vi "4155C Make Big 2d array FPP.vi"(0 "1D Var1":dbl[](array[numeric])=[0.0, 1.0, 2.0, 3.0, 4.0, 5.0, 6.0, 7.0, 8.0, 9.0, 10.0, 11.0] format="%.2f", 2 "1d ID":dbl[](array[numeric])=[20.0, 21.0, 22.0, 23.0, 24.0, 25.0, 26.0, 27.0, 28.0, 29.0, 30.0, 31.0] format="%.2f", 3 "1d Vp2":dbl[](array[numeric])=[20.0, 21.0, 22.0, 23.0, 24.0, 25.0, 26.0, 27.0, 28.0, 29.0, 30.0, 31.0] format="%.2f", 4 "1d IG":dbl[](array[numeric])=[40.0, 41.0, 42.0, 43.0, 44.0, 45.0, 46.0, 47.0, 48.0, 49.0, 50.0, 51.0] format="%.2f", 6 "1d Vp1":dbl[](array[numeric])=[60.0, 61.0, 62.0, 63.0, 64.0, 65.0, 66.0, 67.0, 68.0, 69.0, 70.0, 71.0] format="%.2f", 10 "VAR2 START":dbl format="%.2f", 11 "Number of VAR2 steps":i32=6, 14 "VAR2 STEP":dbl format="%.2f", 15 "VAR1 Name":string, 24 "Decimal places in header":i8=1, 26 "VAR2 Name":string) -> (20 "Header array":string[](array[string]), 22 "Data array":dbl[][](array[numeric]) format="%.2f")   [LabVIEW 2019]
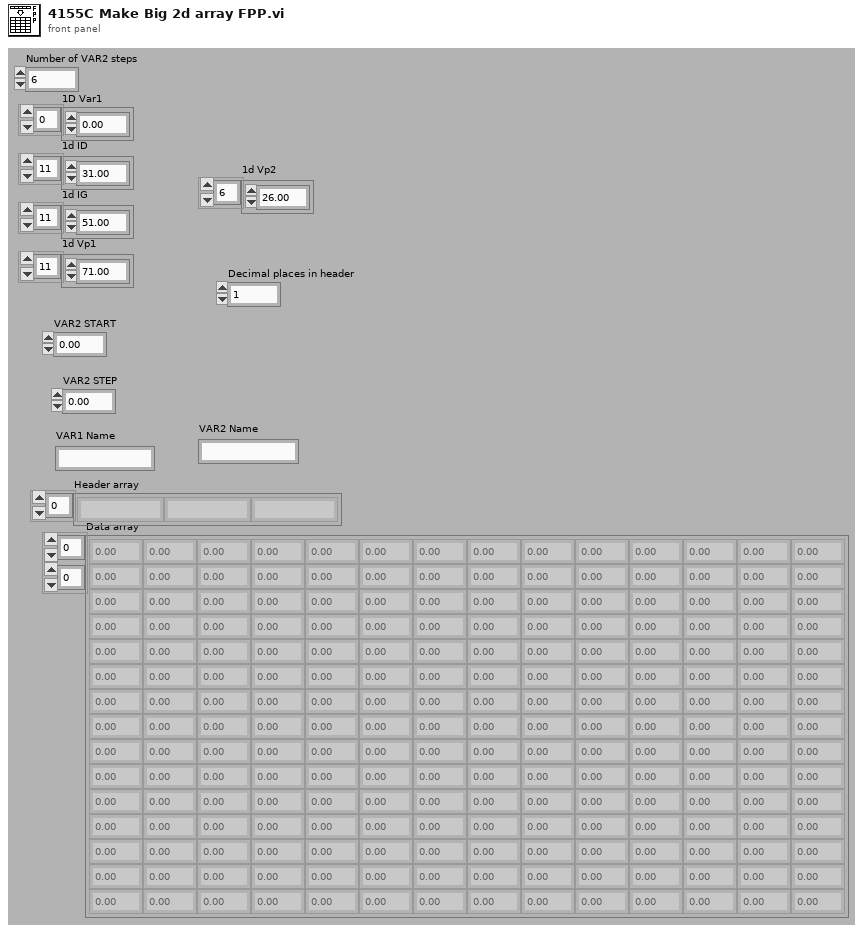
[diagram p1: front panel]
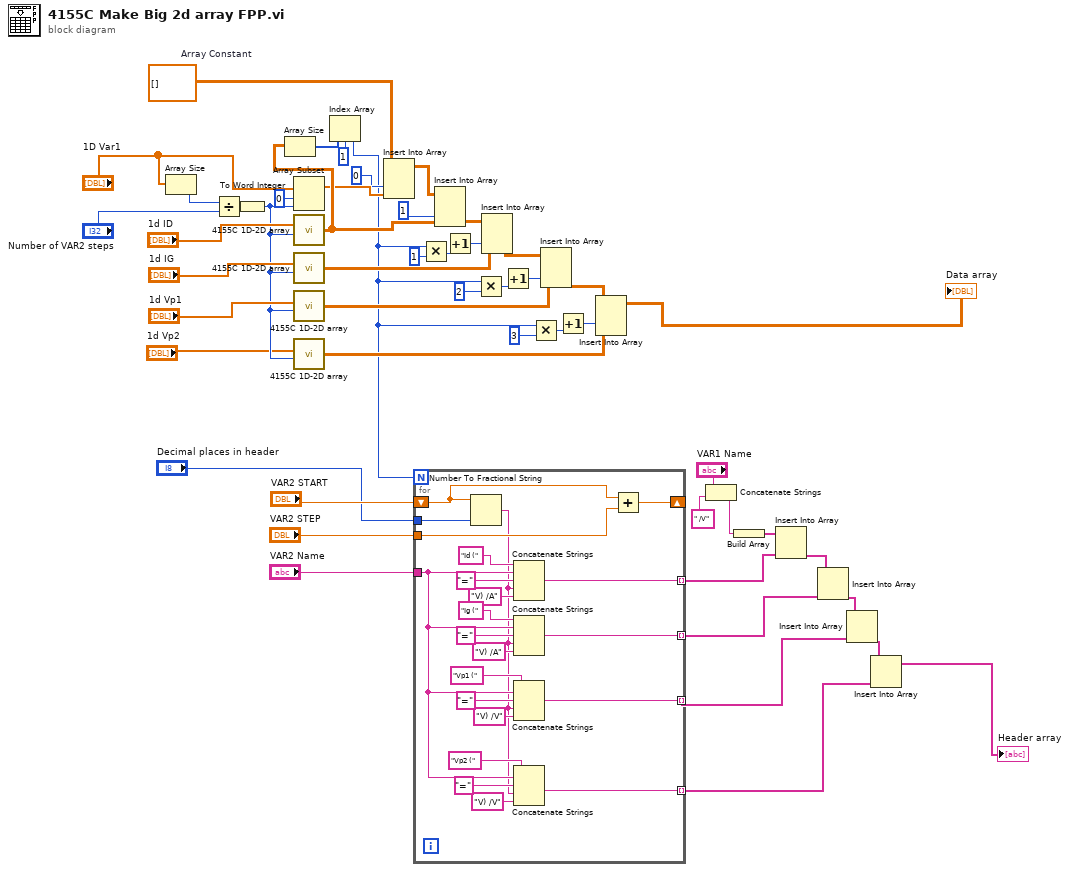
[diagram p0: block diagram]
diagram:
  w37 = dbl[][] []  # Array Constant
  n1 = Array Size(array="1D Var1") -> (size(s)=w14:i32)
  n2 = Divide(x=w14, y="Number of VAR2 steps") -> (x/y=w16:dbl)
  n3 = To Word Integer(number=w16) -> (16bit integer=w8:i16)
  n4 = Array Subset(array="1D Var1", index=0 ("Array Index"), length=w8) -> (w36:dbl[])
  n5 = call "4155C 1D-2D array.vi"("Number of VAR1 steps"=w8, "1D array in"="1d ID") -> ("2D array out"=w43:dbl[][])  [unwired: 4 in]
  n6 = Array Size(array=w43) -> (size(s)=w51:i32[])
  n7 = call "4155C 1D-2D array.vi"("Number of VAR1 steps"=w8, "1D array in"="1d IG") -> ("2D array out"=w47:dbl[][])  [unwired: 4 in]
  n8 = call "4155C 1D-2D array.vi"("Number of VAR1 steps"=w8, "1D array in"="1d Vp1") -> ("2D array out"=w44:dbl[][])  [unwired: 4 in]
  n9 = call "4155C 1D-2D array.vi"("Number of VAR1 steps"=w8, "1D array in"="1d Vp2") -> ("2D array out"=w11:dbl[][])  [unwired: 4 in]
  n10 = Index Array(array=w51, index=1 ("Index")) -> (element=w3:i32)
  n11 = Insert Into Array(array=w37, index (col)=0 ("Disabled Index (col)"), new element=w36) -> (w38:dbl[][])  [unwired: 1 in]
  n12 = for {
    N: w3 -> [_]
    shift-right: [w73] -> _
    shift-left: "VAR2 START" -> [w72]
    tunnel: "VAR2 STEP" -> [w71]
    tunnel: "VAR2 Name" -> [w54]
    tunnel: [w68] -> w25 mode=indexing
    tunnel: [w61] -> w21 mode=indexing
    tunnel: [w60] -> w22 mode=indexing
    tunnel: "Decimal places in header" -> [w58]
    tunnel: [w52] -> w4 mode=indexing
    n13 = Number To Fractional String(number=w72, precision (6)=w58) -> (F-format string=w53:string)  [unwired: 2 in]
    n14 = Concatenate Strings("Id (" ("Substring"), w54, "=" ("Substring"), w53, "V) /A" ("Substring")) -> (w68:string)
    n15 = Concatenate Strings("Ig (" ("Substring"), w54, "=" ("Substring"), w53, "V) /A" ("Substring")) -> (w61:string)
    n16 = Concatenate Strings("Vp1 (" ("Substring"), w54, "=" ("Substring"), w53, "V) /V" ("Substring")) -> (w60:string)
    n17 = Concatenate Strings("Vp2 (" ("Substring"), w54, "=" ("Substring"), w53, "V) /V" ("Substring")) -> (w52:string)
    n18 = Add(x=w72, y=w71) -> (x+y=w73:dbl)
  }
  n19 = Multiply(x=w3, y=1) -> (x*y=w32:i32)
  n20 = Insert Into Array(array=w38, index (col)=1 ("Disabled Index (col)"), new element=w43) -> (w46:dbl[][])  [unwired: 1 in]
  n21 = Increment(x=w32) -> (x+1=w31:i32)
  n22 = Multiply(x=w3, y=2) -> (x*y=w33:i32)
  n23 = Insert Into Array(array=w46, index (col)=w31, new element=w47) -> (w45:dbl[][])  [unwired: 1 in]
  n24 = Increment(x=w33) -> (x+1=w30:i32)
  n25 = Multiply(x=w3, y=3) -> (x*y=w12:i32)
  n26 = Insert Into Array(array=w45, index (col)=w30, new element=w44) -> (w9:dbl[][])  [unwired: 1 in]
  n27 = Increment(x=w12) -> (x+1=w6:i32)
  n28 = Insert Into Array(array=w9, index (col)=w6, new element=w11) -> (→"Data array":dbl[][])  [unwired: 1 in]
  n29 = Concatenate Strings("VAR1 Name", " /V" ("Substring")) -> (w20:string)
  n30 = Build Array(w20) -> (w26:string[])
  n31 = Insert Into Array(array=w26, new element=w25) -> (w24:string[])  [unwired: 1 in]
  n32 = Insert Into Array(array=w24, new element=w21) -> (w23:string[])  [unwired: 1 in]
  n33 = Insert Into Array(array=w23, new element=w22) -> (w5:string[])  [unwired: 1 in]
  n34 = Insert Into Array(array=w5, new element=w4) -> (→"Header array":string[])  [unwired: 1 in]
